vi "matrici_v0_v44.vi"() -> ()   [LabVIEW 2009]
uses:
  <vilib>/Native 3D Graph/xcontrol/3DPC_SurfacePlot.xctl
  <vilib>/Native 3D Graph/classes/Line/Line.lvclass
panel:
  in  "Domeniul de definitie y":dbl(slide)=0.5242070116861437 scale=-2.0..2.0
  out "3D Graph":refnum<class "Base Datatype.lvclass">[](xcontrol)
  out "X":dbl=3.390233722871455
  out "y":dbl=-3.1847650123943945
  in  "stop":bool
  in  "Domeniul de definitie x,y":dbl(slide)=6.780467445742905 scale=0.5..10.0
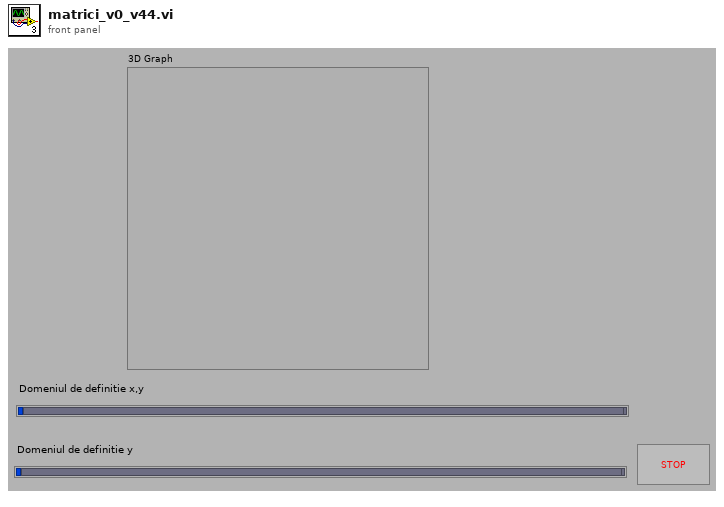
[diagram p1: front panel]
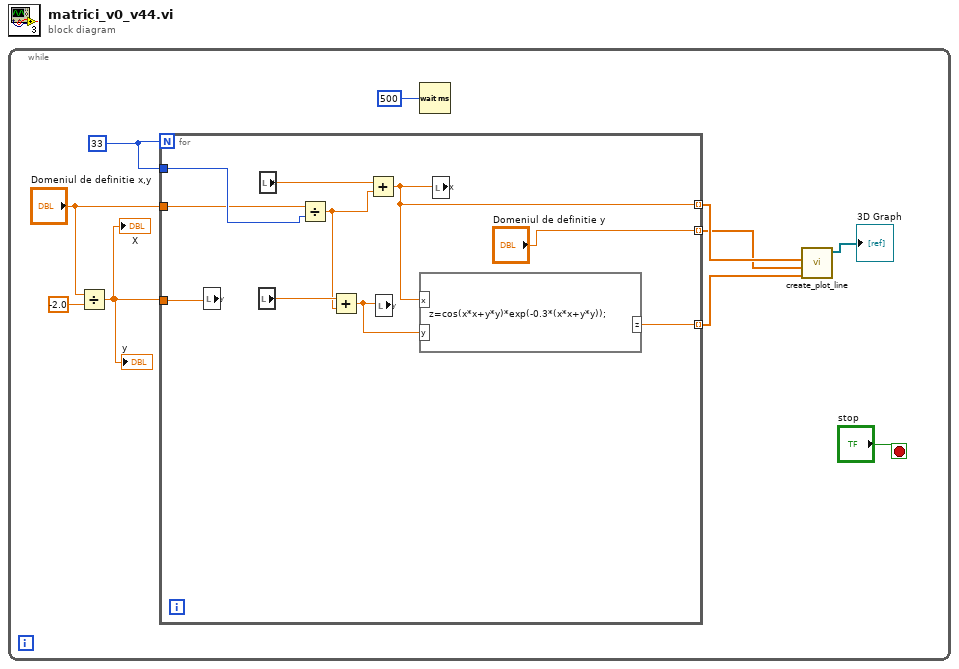
[diagram p0: block diagram]
diagram:
  n1 = while {
    stop <- "stop" stop-if-true
    w8 = 33
    n2 = Divide(x="Domeniul de definitie x,y", y=-2.0) -> (x/y=w5:dbl)
    "X" <- w5
    "y" <- w5
    n3 = for {
      N: w8 -> [_]
      tunnel: [w14] -> w3 mode=indexing
      tunnel: w8 -> [w19]
      tunnel: w5 -> [w18]
      tunnel: "Domeniul de definitie x,y" -> [w17]
      tunnel: [w13] -> w1 mode=indexing
      tunnel: ["Domeniul de definitie y"] -> w2 mode=indexing
      n4 = local write "y"(w18) -> ()
      n5 = local read "y"() -> (w16:dbl)
      n6 = local read "X"() -> (w20:dbl)
      n7 = Divide(x=w17, y=w19) -> (x/y=w15:dbl)
      n8 = Add(x=w16, y=w15) -> (x+y=w12:dbl)
      n9 = Add(x=w20, y=w15) -> (x+y=w14:dbl)
      n10 = local write "y"(w12) -> ()
      n11 = formula code="z=cos(x*x+y*y)*exp(-0.3*(x*x+y*y));"("x"=w14, "y"=w12) -> ("z"=w13:dbl)
      n12 = local write "X"(w14) -> ()
    }
    n13 = Wait (ms)(milliseconds to wait=500) -> ()  [unwired: 1 out]
    n14 = call <vilib>:"create_plot_line.vi"("z vector"=w1, "y vector"=w2, "x vector"=w3) -> ("plots out"=→"3D Graph":refnum<class "Base Datatype.lvclass">[])  [unwired: 2 in, 6 out]
  }
